vi "Birth Date To Birthday.vi"(11 "Birth Date":timestamp) -> (3 "Birthday":timestamp)   [LabVIEW 2019]
doc: "This VI zeroes out the seconds/minutes/hours information of a timestamp and sets the year to 2000 so that all that is left is the birthday information."
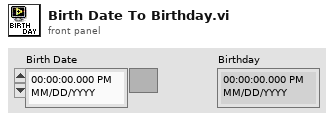
[diagram p1: front panel]
types:
  T1 = typedef "LVDateTimeRec.ctl" = cluster{"fractional second":dbl, "second":i32, "minute":i32, "hour":i32, "day of month":i32, "month":i32, "year":i32, "day of week":i32, "day of year":i32, "DST":i32}
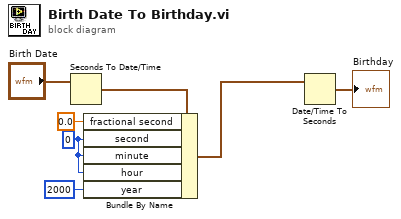
[diagram p0: block diagram]
diagram:
  w4 = 0 ("second")
  n1 = Seconds To Date/Time(time stamp (now)="Birth Date") -> (date time rec=w6:T1)  [unwired: 1 in]
  n2 = Bundle By Name(cluster=w6, "fractional second"=0.0, "second"=w4, "minute"=w4, "hour"=w4, "year"=2000) -> (w2:T1)
  n3 = Date/Time To Seconds(2:w2) -> (0:→"Birthday":timestamp)  [unwired: 1 in]
